vi "Restrict window size(s).vi"(6 "Disable in":bool, 7 "Function":T1(ring)=enum."Prevent all resizing", 10 "Window size":cluster{"Horisontal":i16, "Vertical":i16}, 11 "VI in":refnum<vi>) -> (3 "VI out":refnum<vi>)   [LabVIEW 2017]
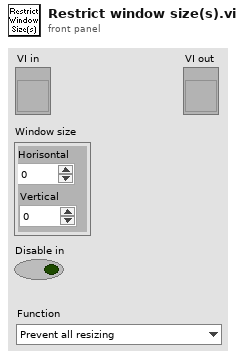
[diagram p1: front panel]
types:
  T1 = enum16{"Prevent horisontal resizing", "Prevent vertical resizing", "Prevent all resizing"}
  T2 = typedef "LVRectTypeDef.ctl" = cluster{"Left":i16, "Top":i16, "Right":i16, "Bottom":i16}
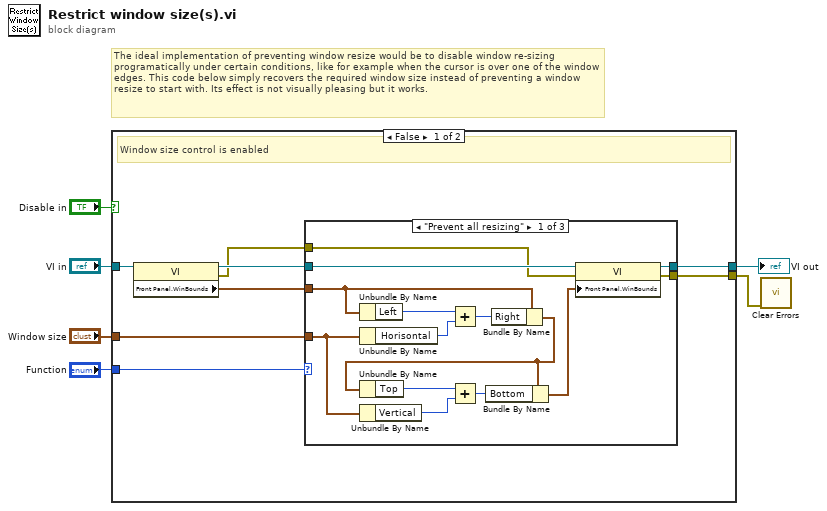
[diagram p0: block diagram]
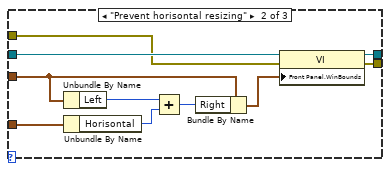
[diagram p2: hidden frame]
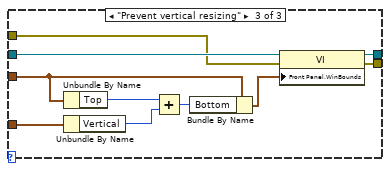
[diagram p3: hidden frame]
diagram:
  # "The ideal implementation of preventing window resize would be to disable window re-sizing programatically under certain conditions, like for example when the cursor is over one of the window edges. This code below simply recovers the required window size instead of preventing a window resize to start with. Its effect is not visually pleasing but it works."
  n1 = case shown="False" "Disable in" {
    tunnel: [w9 w49] -> w6
    tunnel: "VI in" -> [w14 w49]
    tunnel: "Window size" -> [w13 _]
    tunnel: "Function" -> [w12 _]
    tunnel: [w7 _] -> w1
    frame False {
      # "Window size control is enabled"
      n2 = property on="Property Node" class="VI"(reference=w14) -> (reference out=w10:refnum<vi>, error out=w8:errorcluster, "Front Panel.WinBounds"=w11:T2)  [unwired: 1 in]
      n3 = case shown="\"Prevent all resizing\"" w12 {
        tunnel: w13 -> [w19 w37 w47]
        tunnel: w11 -> [w20 w35 w45]
        tunnel: w10 -> [w25 w32 w42]
        tunnel: [w24 w31 w41] -> w9
        tunnel: [w15 w30 w39] -> w7
        tunnel: w8 -> [w16 w29 w40]
        frame "Prevent all resizing" {
          n4 = Unbundle By Name(w20) -> ("Left"=w28:i16)
          n5 = Unbundle By Name(w19) -> ("Horisontal"=w27:i16)
          n6 = Unbundle By Name(w19) -> ("Vertical"=w22:i16)
          n7 = Add(x=w28, y=w27) -> (x+y=w26:i16)
          n8 = Bundle By Name(cluster=w20, "Right"=w26) -> (w18:T2)
          n9 = Unbundle By Name(w18) -> ("Top"=w23:i16)
          n10 = Add(x=w23, y=w22) -> (x+y=w21:i16)
          n11 = Bundle By Name(cluster=w18, "Bottom"=w21) -> (w17:T2)
          n12 = property on="Property Node" class="VI"(reference=w25, error in=w16, "Front Panel.WinBounds"=w17) -> (reference out=w24:refnum<vi>, error out=w15:errorcluster)
        }
        frame "Prevent horisontal resizing" {
          n13 = Unbundle By Name(w35) -> ("Left"=w38:i16)
          n14 = Unbundle By Name(w37) -> ("Horisontal"=w36:i16)
          n15 = Add(x=w38, y=w36) -> (x+y=w34:i16)
          n16 = Bundle By Name(cluster=w35, "Right"=w34) -> (w33:T2)
          n17 = property on="Property Node" class="VI"(reference=w32, error in=w29, "Front Panel.WinBounds"=w33) -> (reference out=w31:refnum<vi>, error out=w30:errorcluster)
        }
        frame "Prevent vertical resizing" {
          n18 = Unbundle By Name(w45) -> ("Top"=w48:i16)
          n19 = Unbundle By Name(w47) -> ("Vertical"=w46:i16)
          n20 = Add(x=w48, y=w46) -> (x+y=w44:i16)
          n21 = Bundle By Name(cluster=w45, "Bottom"=w44) -> (w43:T2)
          n22 = property on="Property Node" class="VI"(reference=w42, error in=w40, "Front Panel.WinBounds"=w43) -> (reference out=w41:refnum<vi>, error out=w39:errorcluster)
        }
      }
    }
    frame True {
      # "Window size control is disabled"
    }
  }
  "VI out" <- w6
  n23 = call <vilib>:"Clear Errors.vi"("error in (no error)"=w1) -> ()  [unwired: 5 in, 2 out]
